vi "SendToDb.vi"(0 "reference in":refnum<class "Engine_1DO_2DI.lvclass">, 11 "error in (no error)":errorcluster) -> (4 "reference out":refnum<class "Engine_1DO_2DI.lvclass">, 15 "error out":errorcluster)   [LabVIEW 2019, in "Engine_1DO_2DI.lvclass"]
uses:
  Engine_1DO_2DI.lvclass
  C:/Users/ANENKOV_V1/Desktop/src/Proccess_class/Proccess.lvclass
  Engine_1DO_2DI.lvclass/Engine_1DO_2DI.ctl
  Proccess_class/Proccess.lvclass/Proccess.ctl
  Logger_class/EventData.ctl
  TypeDef/AlarmType.ctl
  c0b53383-3d34-4a55-8dce-306f7f934b6c.vi
  Logger_class/Logger.lvclass
  Proccess_class/Proccess.lvclass
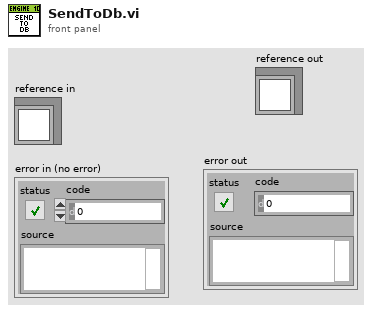
[diagram p1: front panel]
types:
  T1 = typedef "State Engine.ctl" = enum16{"Unknown", "Off", "TupningOn", "On", "TurningOff"}
  T2 = typedef "EventData.ctl" = cluster{"obj_tag":string, "event_tag":string, "Description":string, "ALARM TYPE":T3, "Value DBL":dbl, "Value INT":i32, "Value STR":string, "Time Stamp":timestamp}
  T3 = typedef "AlarmType.ctl" = enum16{"Normal", "Warning", "Alarm"}
  T4 = typedef "Proccess.lvclass/TAGs.ctl" = cluster{"TAG":string, "PTAG":string, "DESC":string}
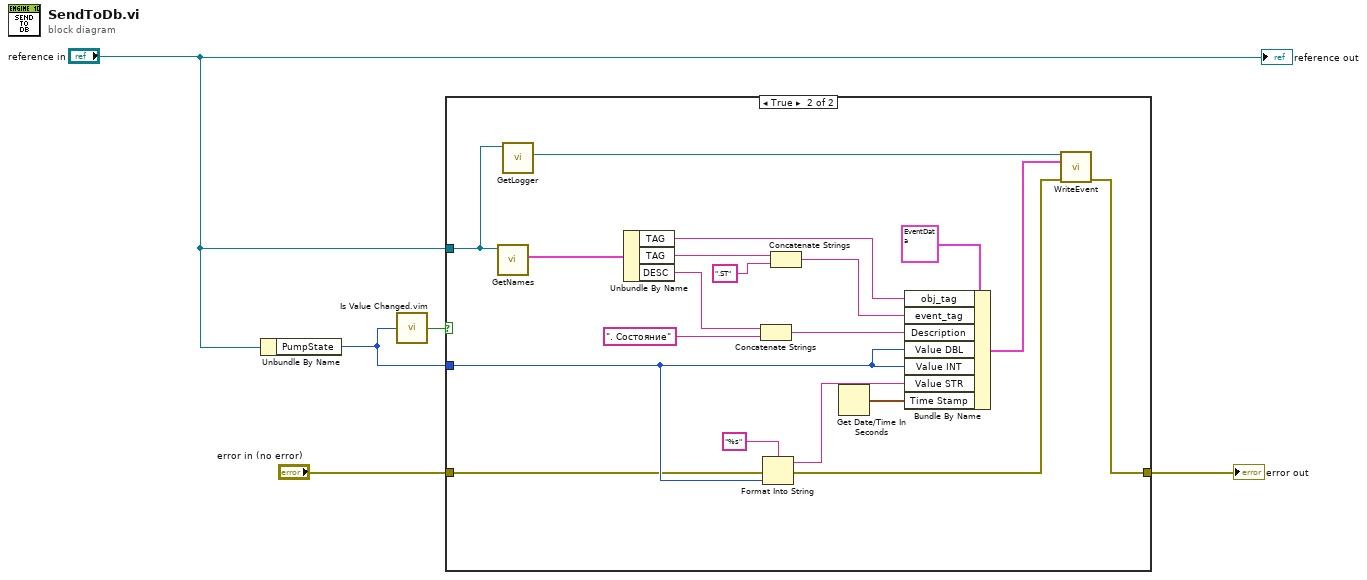
[diagram p0: block diagram]
diagram:
  n1 = Unbundle By Name("reference in") -> ("PumpState"=w2:T1)
  n2 = call "Is Value Changed.vim"("value"=w2) -> ("changed or first call?"=w1:bool)
  n3 = case shown="True" w1 {
    tunnel: [w6 w25] -> w5
    tunnel: "reference in" -> [_ w19]
    tunnel: w2 -> [_ w12]
    tunnel: "error in (no error)" -> [w6 w10]
    frame False {
    }
    frame True {
      n4 = call "GetNames.vi"("Proccess in"=w19) -> ("Tags"=w18:T4)  [unwired: 10 in]
      n5 = call "GetLogger.vi"("Proccess in"=w19) -> ("Logger"=w20:refnum<class "Logger.lvclass">)  [unwired: 10 in]
      n6 = Unbundle By Name(w18) -> ("TAG"=w17:string, "TAG"=w16:string, "DESC"=w15:string)
      n7 = Concatenate Strings(w15, ". Состояние" ("string")) -> (w8:string)
      n8 = Format Into String(format string="%s", error in=w10, w12) -> (resulting string=w11:string, error out=w9:errorcluster)  [unwired: 1 in]
      n9 = Concatenate Strings(w16, ".ST" ("string")) -> (w22:string)
      n10 = Get Date/Time In Seconds() -> (seconds since 1Jan1904=w14:timestamp)
      n11 = Bundle By Name(cluster=T2 {"obj_tag"="", "event_tag"="", "Description"="", "ALARM TYPE"=enum."Normal", "Value DBL"=0.0, "Value INT"=0, "Value STR"="", "Time Stamp"=timestamp(0 s since 1904-01-01)} ("Event"), "obj_tag"=w17, "event_tag"=w22, "Description"=w8, "Value DBL"=w12, "Value INT"=w12, "Value STR"=w11, "Time Stamp"=w14) -> (w24:T2)
      n12 = call "WriteEvent.vi"("reference in"=w20, "Event"=w24, "error in (no error)"=w9) -> ("error out"=w25:errorcluster)  [unwired: 11 in, 1 out]
    }
  }
  "error out" <- w5
  "reference out" <- "reference in"
